vi "test.parse.fields.vi"() -> (3 "All Passed":bool)   [LabVIEW 2022 SP3]
uses:
  parse.field.test.case.ctl
  <vilib>/rvi/Emulation/niFpgaGetClockAttributes.vi
  <vilib>/rvi/Emulation/niFpgaSctlEmulationGetInTimedLoop.vi
  <vilib>/rvi/Emulation/niFpgaEmulationReportErrorSimple.vi
  <vilib>/rvi/Emulation/niFpgaCriticalErrorInLSC.vi
panel:
  out "Passed 5":bool
  in  "Test Case #5 - Length of 8, across 2 WORDS 3 bytes spill":T1={"buffer.length"=8, "start.idx"=19, "buffer"=[2459274161843883858, 5279397646710161952, 5620492615227034656, 2331214240024625152, 281474976710656, 0, 0, 0, 0], "U8"=FALSE, "exp.u8"=0, "U16"=FALSE, "exp.u16"=0, "U32"=FALSE, "exp.u32"=0, "U64"=TRUE, "exp.u64"=2547383862322807105} {"exp.u64" format="%.0x"; "exp.u32" format="%.0x"; "exp.u16" format="%.0x"; "exp.u8" format="%.0x"; "buffer" format="%016x"}
  out "Passed 4":bool
  in  "Test Case #4 - Ticker - Length of 6, across 2 WORDS 3 bytes spill":T1={"buffer.length"=6, "start.idx"=19, "buffer"=[2459274161843883858, 5279397646710161952, 5620492615227034656, 2331214240024625152, 281474976710656, 0, 0, 0, 0], "U8"=FALSE, "exp.u8"=0, "U16"=FALSE, "exp.u16"=0, "U32"=FALSE, "exp.u32"=0, "U64"=TRUE, "exp.u64"=4702127773838221344} {"exp.u64" format="%.0x"; "exp.u32" format="%.0x"; "exp.u16" format="%.0x"; "exp.u8" format="%.0x"; "buffer" format="%016x"}
  out "Passed 3":bool
  in  "Test Case #3 - Ticker - Length of 6, across 2 WORDS 2 bytes spill":T1={"buffer.length"=6, "start.idx"=19, "buffer"=[2459274161843883858, 5279397646710161952, 5620492615227034656, 2331214240024625152, 281474976710656, 0, 0, 0, 0], "U8"=FALSE, "exp.u8"=0, "U16"=FALSE, "exp.u16"=0, "U32"=FALSE, "exp.u32"=0, "U64"=TRUE, "exp.u64"=4702127773838221344} {"exp.u64" format="%.0x"; "exp.u32" format="%.0x"; "exp.u16" format="%.0x"; "exp.u8" format="%.0x"; "buffer" format="%016x"}
  out "Passed 2":bool
  in  "Test Case #2 - Ticker - Length of 6, across 2 WORDS 1 byte spill":T1={"buffer.length"=6, "start.idx"=19, "buffer"=[2459274161843883858, 5279397646710161952, 5620492615227034656, 2331214240024625152, 281474976710656, 0, 0, 0, 0], "U8"=FALSE, "exp.u8"=0, "U16"=FALSE, "exp.u16"=0, "U32"=FALSE, "exp.u32"=0, "U64"=TRUE, "exp.u64"=4702127773838221344} {"exp.u64" format="%.0x"; "exp.u32" format="%.0x"; "exp.u16" format="%.0x"; "exp.u8" format="%.0x"; "buffer" format="%016x"}
  in  "Test Case #1 - Sequenced Unit Header - Hdr Length":T1={"buffer.length"=8, "start.idx"=0, "buffer"=[3026420053433122816, 0, 0, 0, 0, 0, 0, 0, 0], "U8"=FALSE, "exp.u8"=0, "U16"=TRUE, "exp.u16"=42, "U32"=FALSE, "exp.u32"=0, "U64"=FALSE, "exp.u64"=0} {"exp.u64" format="%.0x"; "exp.u32" format="%.0x"; "exp.u16" format="%.0x"; "exp.u8" format="%.0x"; "buffer" format="%016x"}
  in  "Test #":i32=1
  in  "Override":bool
  out "Passed 1":bool
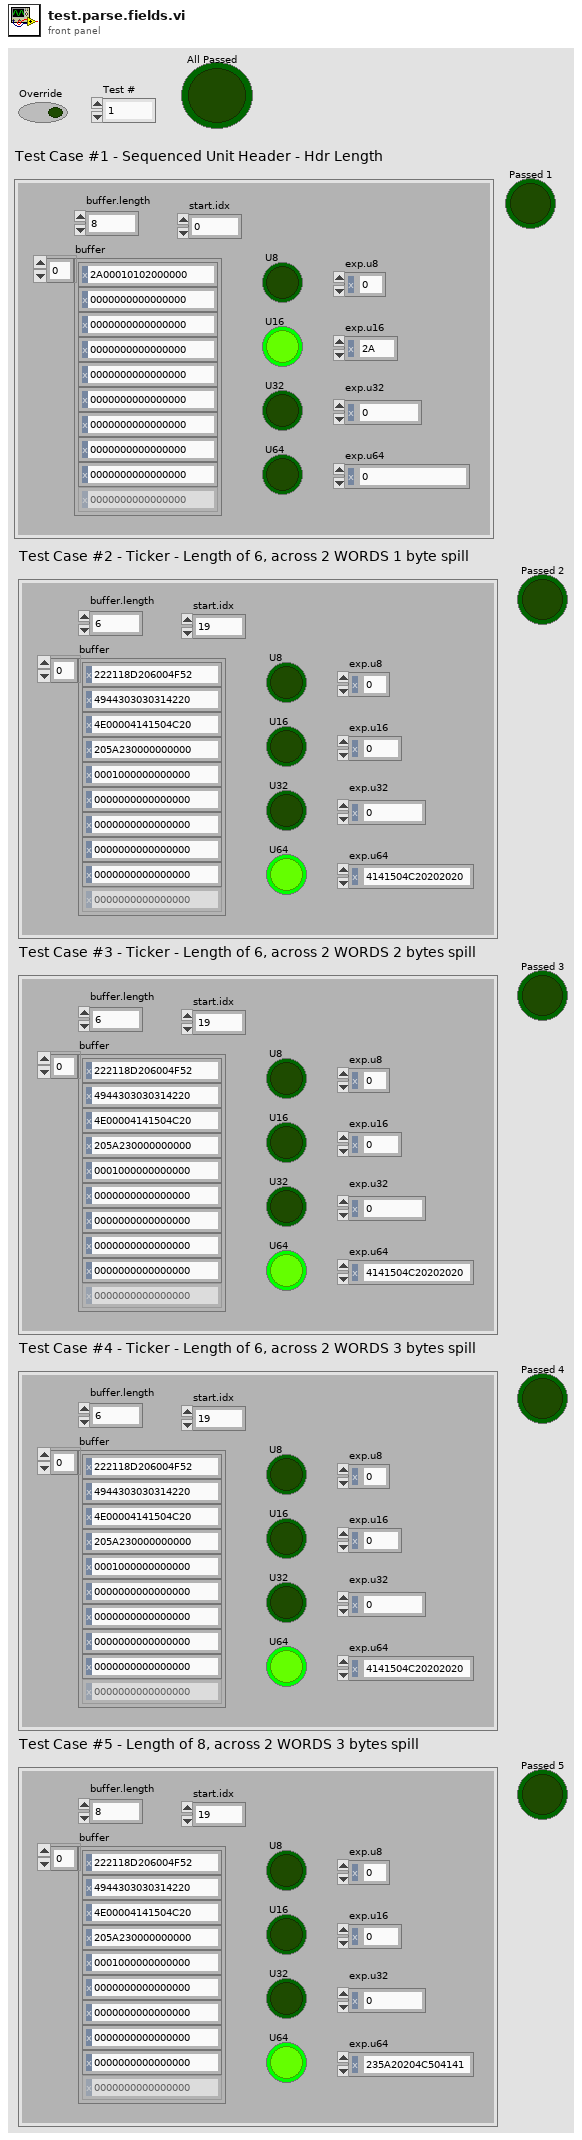
[diagram p1: front panel]
types:
  T1 = typedef "parse.field.test.case.ctl" = cluster{"buffer.length":u8, "start.idx":u8, "buffer":u64[], "U8":bool, "exp.u8":u8, "U16":bool, "exp.u16":u16, "U32":bool, "exp.u32":u32, "U64":bool, "exp.u64":u64}
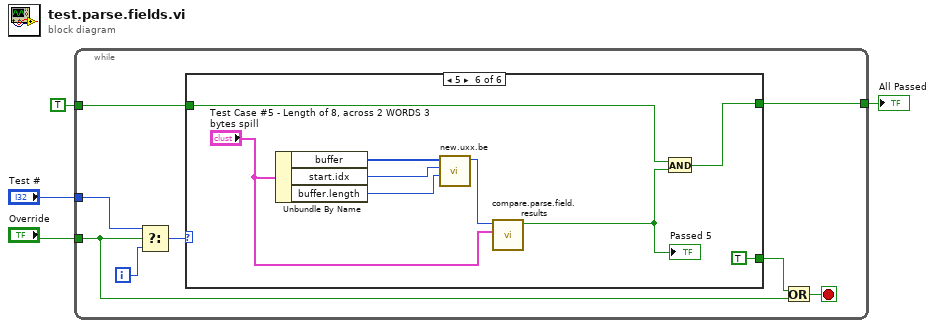
[diagram p0: block diagram]
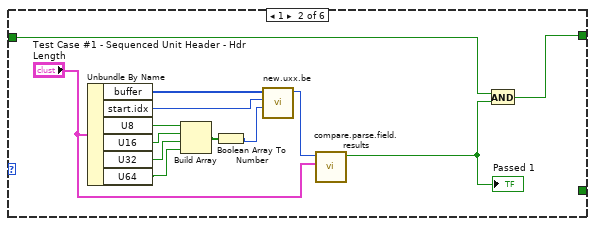
[diagram p3: hidden frame]
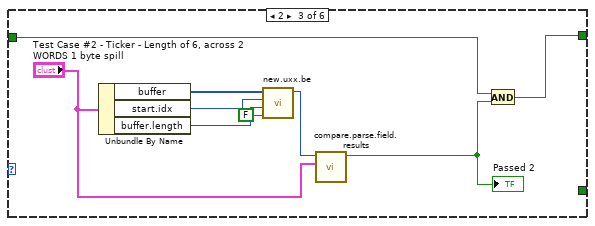
[diagram p4: hidden frame]
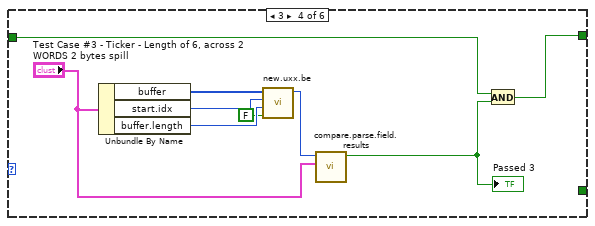
[diagram p5: hidden frame]
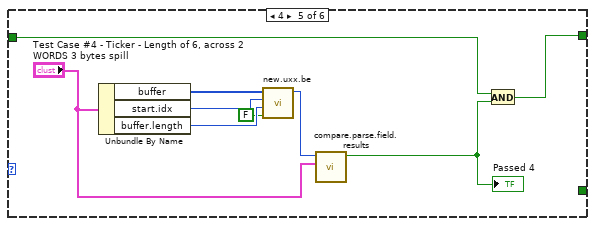
[diagram p6: hidden frame]
diagram:
  n1 = while {
    tunnel: TRUE -> [w11]
    tunnel: [w10] -> w1
    tunnel: "Test #" -> [w9]
    tunnel: "Override" -> [w5]
    i -> [w8]
    stop <- w6 stop-if-true
    n2 = Select(t=w9, s=w5, f=w8) -> (s? t:f=w7:i32)
    n3 = case shown="5" w7 {
      tunnel: [_ _ _ _ _ TRUE] -> w12
      tunnel: w11 -> [w13 w25 w34 w43 w52 w61]
      tunnel: [w13 w26 w35 w44 w53 w62] -> w10
      frame 0, Default {
      }
      frame 1 {
        n4 = Unbundle By Name("Test Case #1 - Sequenced Unit Header - Hdr Length") -> ("buffer"=w17:u64[], "start.idx"=w16:u8, "U8"=w22:bool, "U16"=w21:bool, "U32"=w20:bool, "U64"=w19:bool)
        n5 = Build Array(w22, w21, w20, w19) -> (w18:bool[])
        n6 = Boolean Array To Number(Boolean array=w18) -> (number=w15:u8)
        n7 = call "new.uxx.be.vi"("buffer (U64)"=w17, "Start.Idx"=w16, "Length"=w15) -> ("Uxx.be"=w14:u64)  [unwired: 7 in]
        n8 = call "compare.parse.field.results.vi"("Test Case #1 - Sequenced Unit Header - Hdr Length"="Test Case #1 - Sequenced Unit Header - Hdr Length", "Val.in"=w14) -> ("Equal?"=w23:bool)  [unwired: 9 in]
        "Passed 1" <- w23
        n9 = And(x=w25, y=w23) -> (x .and. y?=w26:bool)
      }
      frame 2 {
        n10 = Unbundle By Name("Test Case #2 - Ticker - Length of 6, across 2 WORDS 1 byte spill") -> ("buffer"=w31:u64[], "start.idx"=w30:u8, "buffer.length"=w28:u8)
        n11 = call "new.uxx.be.vi"("buffer (U64)"=w31, "Start.Idx"=w30, "Length"=w28, "Big.Endian?"=FALSE) -> ("Uxx.be"=w29:u64)  [unwired: 6 in]
        n12 = call "compare.parse.field.results.vi"("Test Case #1 - Sequenced Unit Header - Hdr Length"="Test Case #2 - Ticker - Length of 6, across 2 WORDS 1 byte spill", "Val.in"=w29) -> ("Equal?"=w32:bool)  [unwired: 9 in]
        "Passed 2" <- w32
        n13 = And(x=w34, y=w32) -> (x .and. y?=w35:bool)
      }
      frame 3 {
        n14 = Unbundle By Name("Test Case #3 - Ticker - Length of 6, across 2 WORDS 2 bytes spill") -> ("buffer"=w40:u64[], "start.idx"=w39:u8, "buffer.length"=w37:u8)
        n15 = call "new.uxx.be.vi"("buffer (U64)"=w40, "Start.Idx"=w39, "Length"=w37, "Big.Endian?"=FALSE) -> ("Uxx.be"=w38:u64)  [unwired: 6 in]
        n16 = call "compare.parse.field.results.vi"("Test Case #1 - Sequenced Unit Header - Hdr Length"="Test Case #3 - Ticker - Length of 6, across 2 WORDS 2 bytes spill", "Val.in"=w38) -> ("Equal?"=w41:bool)  [unwired: 9 in]
        "Passed 3" <- w41
        n17 = And(x=w43, y=w41) -> (x .and. y?=w44:bool)
      }
      frame 4 {
        n18 = Unbundle By Name("Test Case #4 - Ticker - Length of 6, across 2 WORDS 3 bytes spill") -> ("buffer"=w49:u64[], "start.idx"=w48:u8, "buffer.length"=w46:u8)
        n19 = call "new.uxx.be.vi"("buffer (U64)"=w49, "Start.Idx"=w48, "Length"=w46, "Big.Endian?"=FALSE) -> ("Uxx.be"=w47:u64)  [unwired: 6 in]
        n20 = call "compare.parse.field.results.vi"("Test Case #1 - Sequenced Unit Header - Hdr Length"="Test Case #4 - Ticker - Length of 6, across 2 WORDS 3 bytes spill", "Val.in"=w47) -> ("Equal?"=w50:bool)  [unwired: 9 in]
        "Passed 4" <- w50
        n21 = And(x=w52, y=w50) -> (x .and. y?=w53:bool)
      }
      frame 5 {
        n22 = Unbundle By Name("Test Case #5 - Length of 8, across 2 WORDS 3 bytes spill") -> ("buffer"=w58:u64[], "start.idx"=w57:u8, "buffer.length"=w55:u8)
        n23 = call "new.uxx.be.vi"("buffer (U64)"=w58, "Start.Idx"=w57, "Length"=w55) -> ("Uxx.be"=w56:u64)  [unwired: 7 in]
        n24 = call "compare.parse.field.results.vi"("Test Case #1 - Sequenced Unit Header - Hdr Length"="Test Case #5 - Length of 8, across 2 WORDS 3 bytes spill", "Val.in"=w56) -> ("Equal?"=w59:bool)  [unwired: 9 in]
        "Passed 5" <- w59
        n25 = And(x=w61, y=w59) -> (x .and. y?=w62:bool)
      }
    }
    n26 = Or(x=w12, y=w5) -> (x .or. y?=w6:bool)
  }
  "All Passed" <- w1
